vi "Extend Digital Pattern Over Cycle.vi"(9 "Rotations":u16, 10 "Pattern":T5, 11 "EPT Pattern":T1) -> (2 "Pattern":T5, 3 "Base Repeats":i32)   [LabVIEW 2020, in "Engine Simulation Toolkit System Explorer.lvlib"]
uses:
  Engine Simulation Toolkit System Explorer.lvlib
  Digital Pattern Expanded.ctl
  Digital Pattern.ctl
  Digital Pattern Base.ctl
  Digital Pattern Remove Edge.ctl
  Digital Pattern Add Pulse.ctl
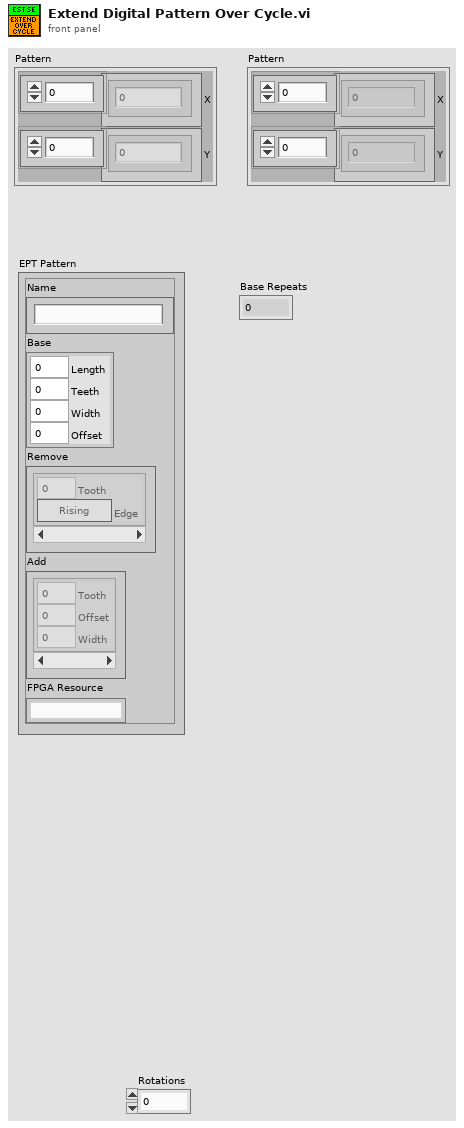
[diagram p1: front panel]
types:
  T1 = typedef "Engine Simulation Toolkit System Explorer.lvlib/Digital Pattern.ctl" = cluster{"Name":string, "Base":T2, "Remove":T3[], "Add":T4[], "FPGA Resource":string}
  T2 = typedef "Engine Simulation Toolkit System Explorer.lvlib/Digital Pattern Base.ctl" = cluster{"Length":dbl, "Teeth":u16, "Width":dbl, "Offset":dbl}
  T3 = typedef "Engine Simulation Toolkit System Explorer.lvlib/Digital Pattern Remove Edge.ctl" = cluster{"Tooth":u16, "Edge":bool}
  T4 = typedef "Engine Simulation Toolkit System Explorer.lvlib/Digital Pattern Add Pulse.ctl" = cluster{"Tooth":u16, "Offset":dbl, "Width":dbl}
  T5 = typedef "Engine Simulation Toolkit System Explorer.lvlib/Digital Pattern Expanded.ctl" = cluster{"X":dbl[], "Y":dbl[]}
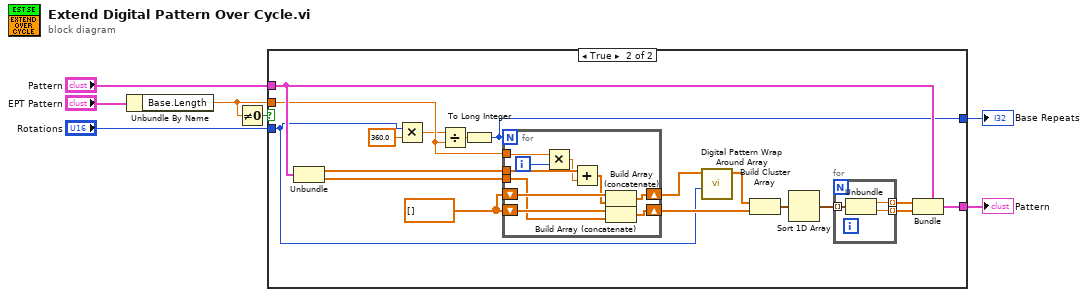
[diagram p0: block diagram]
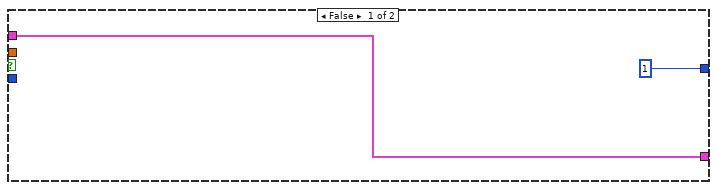
[diagram p2: hidden frame]
diagram:
  n1 = Unbundle By Name("EPT Pattern") -> ("Base.Length"=w2:dbl)
  n2 = Not Equal To 0?(x=w2) -> (x != 0?=w3:bool)
  n3 = case shown="True" w3 {
    tunnel: [w9 w27] -> w7
    tunnel: "Rotations" -> [_ w12]
    tunnel: "Pattern" -> [w9 w26]
    tunnel: w2 -> [_ w18]
    tunnel: [1 w10] -> w1
    frame False {
    }
    frame True {
      w17 = dbl[] []
      n4 = Unbundle(w26) -> ("X"=w15:dbl[], "Y"=w16:dbl[])
      n5 = Multiply(x=w12, y=360.0) -> (x*y=w14:dbl)
      n6 = Divide(x=w14, y=w18) -> (x/y=w11:dbl)
      n7 = To Long Integer(number=w11) -> (32bit integer=w10:i32)
      n8 = for {
        N: w10 -> [_]
        shift-right: [w39] -> w21
        shift-left: w17 -> [w40]
        shift-right: [w37] -> w23
        shift-left: w17 -> [w38]
        tunnel: w15 -> [w35]
        tunnel: w16 -> [w36]
        tunnel: w18 -> [w32]
        i -> [w31]
        n9 = Multiply(x=w32, y=w31) -> (x*y=w33:dbl)
        n10 = Add(x=w35, y=w33) -> (x+y=w34:dbl[])
        n11 = Build Array (concatenate)(w40, w34) -> (w39:dbl[])
        n12 = Build Array (concatenate)(w38, w36) -> (w37:dbl[])
      }
      n13 = call "Digital Pattern Wrap Around Array.vi"("Rotations"=w12, "x"=w21) -> ("x"=w20:dbl[])  [unwired: 9 in]
      n14 = Build Cluster Array(w20, w23) -> (w19:cluster{dbl, "Numeric Control":dbl}[])
      n15 = Sort 1D Array(array=w19) -> (sorted array=w22:cluster{dbl, "Numeric Control":dbl}[])
      n16 = for {
        tunnel: w22 -> [w30] mode=indexing
        tunnel: [w29] -> w24 mode=indexing
        tunnel: [w28] -> w25 mode=indexing
        n17 = Unbundle(w30) -> (w29:dbl, "Numeric Control"=w28:dbl)
      }
      n18 = Bundle(cluster=w26, "X"=w24, "Y"=w25) -> (w27:T5)
    }
  }
  "Pattern" <- w7
  "Base Repeats" <- w1
